vi "浮点CDAB转换COD.vi"(11 "数组":i16[](array[numeric]) format="%04xH") -> (3 "数组 2":sgl[](array[numeric]) format="%#.2f")   [LabVIEW 2016, in "斯坦道CODMn.lvlib"]
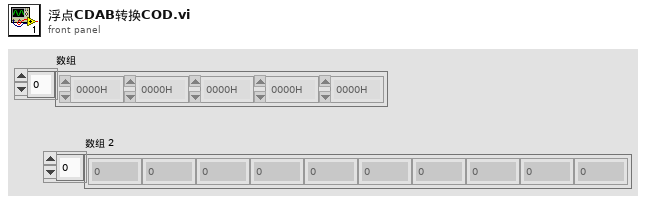
[diagram p1: front panel]
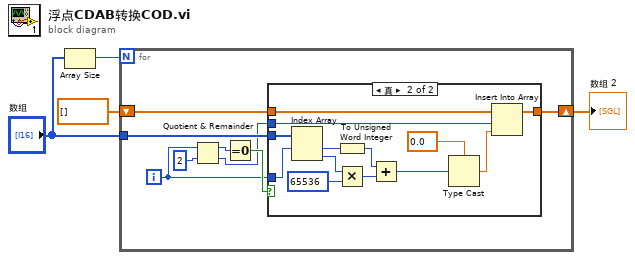
[diagram p0: block diagram]
diagram:
  n1 = Array Size(array="数组") -> (size(s)=w3:i32)
  n2 = for {
    N: w3 -> [_]
    tunnel: "数组" -> [w10]
    shift-right: [w6] -> w2
    shift-left: sgl[] [] ("数组 2") -> [w5]
    i -> [w9]
    n3 = Quotient & Remainder(x=w9, y=2) -> (x-y*floor(x/y)=w7:i32, floor(x/y)=w8:i32)
    n4 = Equal To 0?(x=w7) -> (x = 0?=w11:bool)
    n5 = case shown="真" w11 {
      tunnel: w10 -> [_ w20]
      tunnel: w9 -> [_ w26]
      tunnel: w8 -> [_ w18]
      tunnel: [w13 w15] -> w6
      tunnel: w5 -> [w13 w14]
      frame False {
      }
      frame True {
        n6 = Index Array(array=w20, index #1=w26) -> (element #1=w17:i16, element #2=w16:i16)  [unwired: 1 in]
        n7 = To Unsigned Word Integer(number=w17) -> (unsigned 16bit integer=w22:u16)
        n8 = Multiply(x=w16, y=u32 65536) -> (x*y=w23:u32)
        n9 = Add ("加")(x=w22, y=w23) -> (x+y=w21:u32)
        n10 = Type Cast(type=sgl 0.0, x=w21) -> (*(type *) &x=w19:sgl)
        n11 = Insert Into Array(array=w14, index=w18, new element=w19) -> (w15:sgl[])
      }
    }
  }
  "数组 2" <- w2
